vi "Capture3D.vi"(5 "error in":errorcluster, 6 "Camera Reference in":refnum<k24>) -> (0 "Frame3D Reference out":refnum<k24>, 1 "UntexturedPointCloud Reference out":refnum<k24>, 2 "DepthMap Reference out":refnum<k24>, 3 "error out":errorcluster, 4 "Camera Reference out":refnum<k24>)   [LabVIEW 2023]
uses:
  C:/Users/mech-mind/Downloads/LabView/MechEyeApiNet.dll
  MechEyeApiNet.dll
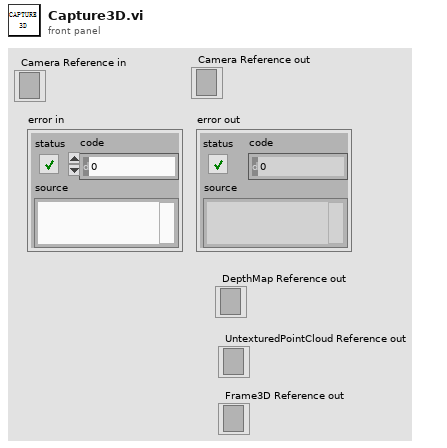
[diagram p1: front panel]
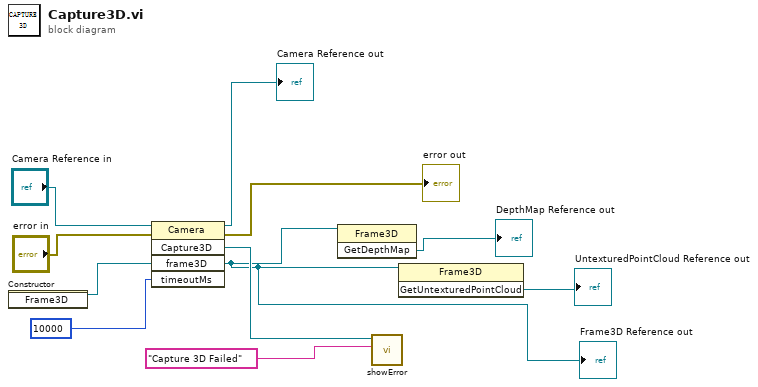
[diagram p0: block diagram]
diagram:
  n1 = constructor class="Frame3D"() -> (reference out=w10:refnum<k24>)  [unwired: 3 in, 2 out]
  n2 = invoke on="Invoke Node" class="Camera" method="Capture3D"(reference="Camera Reference in", error in="error in", "frame3D"=w10, "timeoutMs"=10000) -> (reference out=→"Camera Reference out":refnum<k24>, error out=→"error out":errorcluster, "Capture3D"=w8:refnum<k24>, "frame3D"=w5:refnum<k24>)  [unwired: 1 in, 1 out]
  "Frame3D Reference out" <- w5
  n3 = invoke class="Frame3D" method="GetDepthMap"(reference=w5) -> ("GetDepthMap"=→"DepthMap Reference out":refnum<k24>)  [unwired: 2 in, 2 out]
  n4 = call "showError.vi"("String"="Capture 3D Failed", "ErrorStatus Refnum in"=w8) -> ()  [unwired: 10 in]
  n5 = invoke class="Frame3D" method="GetUntexturedPointCloud"(reference=w5) -> ("GetUntexturedPointCloud"=→"UntexturedPointCloud Reference out":refnum<k24>)  [unwired: 2 in, 2 out]
